vi "SMR_LabVIEW_V2.vi"() -> ()   [LabVIEW 2025]
uses:
  <vilib>/DAQmx/read.llb/DAQmx Read (Analog 1D DBL NChan 1Samp).vi
  <vilib>/Analysis/baseanly.llb/Mean (DBL).vi
  <vilib>/DAQmx/create/channels.llb/DAQmx Create Channel (AI-Temperature-Thermocouple).vi
  <vilib>/DAQmx/create/channels.llb/DAQmx Create Channel (AI-Voltage-Basic).vi
  <vilib>/DAQmx/miscellaneous.llb/DAQmx Fill In Error Info.vi
  <vilib>/Analysis/NI_AALBase.lvlib
panel:
  out "Raw NI9201 \nVoltage Display":T1
  out "Temperature Display":T2
  out "Pressure Display":T3
  in  "Flow Offset Correction (GPM)":dbl=-0.3
  out "Flow History":dbl(graph)
  out "Pressure History":T4(graph)
  out "Temperature History":T5(graph)
  out "Max Loop Pressure (psi)":dbl
  out "Average Loop Temp (deg C)":dbl
  out "Max Loop Temp (deg C)":dbl
  out "Heat Exchanger Flow (GPM)":dbl
  in  "Loop Period (ms)":dbl=1000.0
  in  "Stop":bool
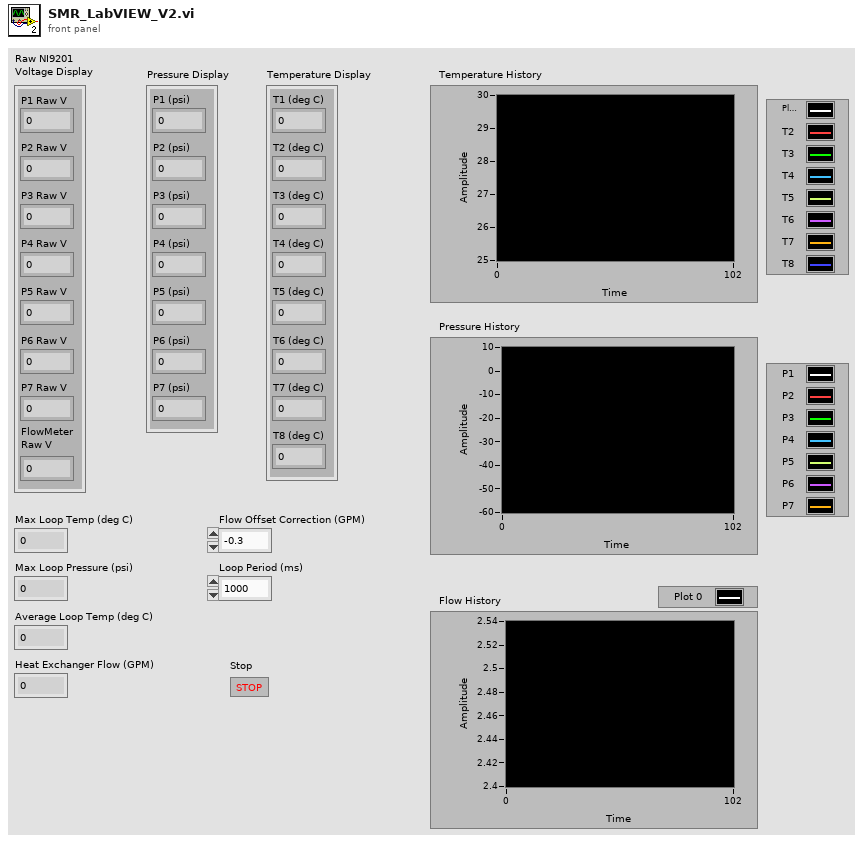
[diagram p1: front panel]
types:
  T1 = cluster{"P1 Raw V":dbl, "P2 Raw V":dbl, "P3 Raw V":dbl, "P4 Raw V":dbl, "P5 Raw V":dbl, "P6 Raw V":dbl, "P7 Raw V":dbl, "FlowMeter\nRaw V":dbl}
  T2 = cluster{"T1 (deg C)":dbl, "T2 (deg C)":dbl, "T3 (deg C)":dbl, "T4 (deg C)":dbl, "T5 (deg C)":dbl, "T6 (deg C)":dbl, "T7 (deg C)":dbl, "T8 (deg C)":dbl}
  T3 = cluster{"P1 (psi)":dbl, "P2 (psi)":dbl, "P3 (psi)":dbl, "P4 (psi)":dbl, "P5 (psi)":dbl, "P6 (psi)":dbl, "P7 (psi)":dbl}
  T4 = cluster{"P1":dbl, "P2":dbl, "P3":dbl, "P4":dbl, "P5":dbl, "P6":dbl, "P7":dbl}
  T5 = cluster{"Waveform":dbl, "Waveform":dbl, "Waveform":dbl, "Waveform":dbl, "Waveform":dbl, "Waveform":dbl, "Waveform":dbl, "Waveform":dbl}
  T6 = cluster{"P1":dbl, "P2":dbl, "P3":dbl, "P4":dbl, "P5":dbl, "P6":dbl, "P7":dbl, "Flow":dbl}
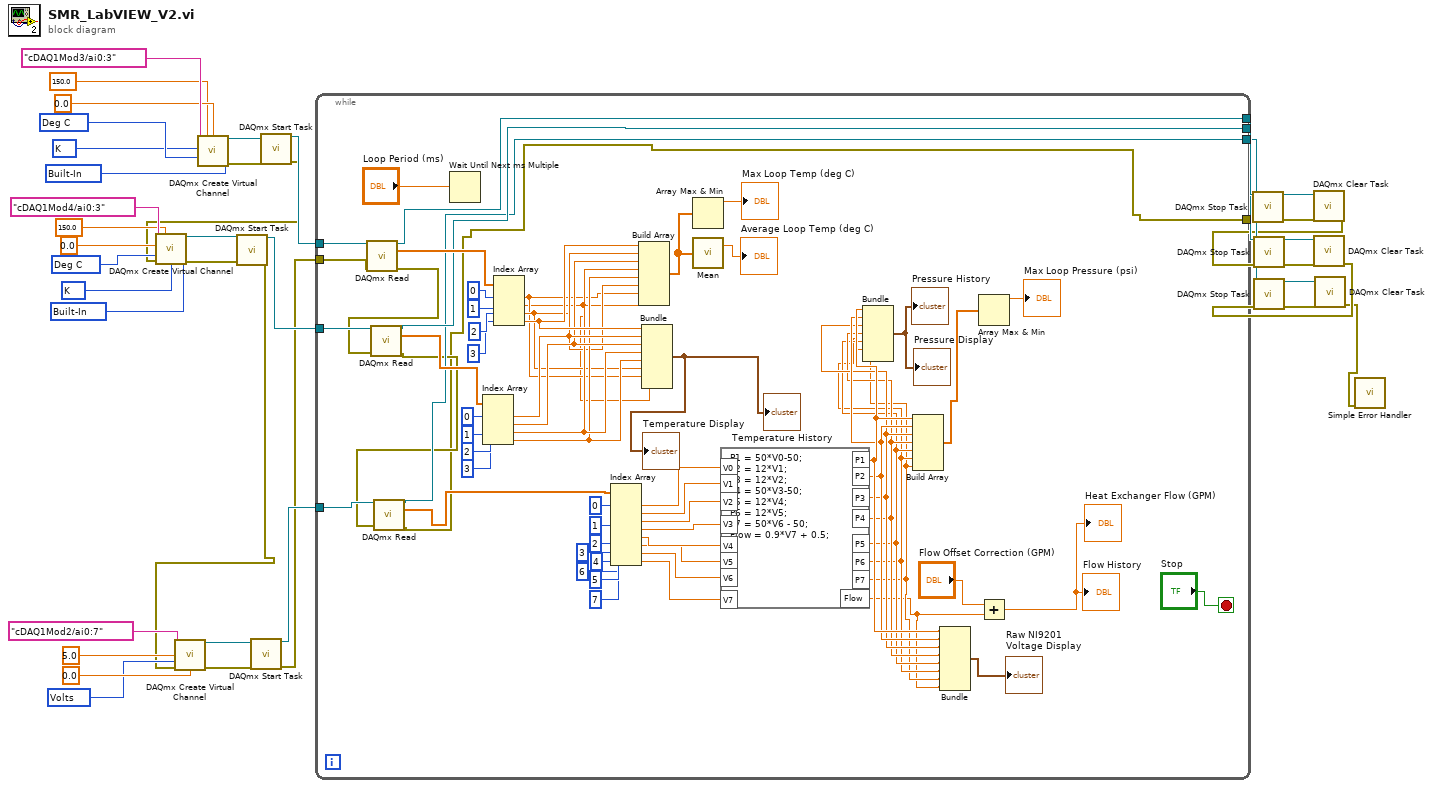
[diagram p0: block diagram]
diagram:
  w23 = 10348 items=["Volts"=10348, "From Custom Scale"=10065] ("units")
  w27 = 10200 items=["Built-In"=10200, "Constant Value"=10116, "Channel"=10113] ("cjc source")
  w28 = 10073 items=["J"=10072, "K"=10073, "N"=10077, "R"=10082, "S"=10085, "T"=10086, "B"=10047, "E"=10055] ("thermocouple type")
  w11 = 10143 items=["Deg C"=10143, "Deg F"=10144, "Kelvins"=10325, "Deg R"=10145, "From Custom Scale"=10065] ("units")
  w31 = 10200 items=["Built-In"=10200, "Constant Value"=10116, "Channel"=10113] ("cjc source")
  w32 = 10073 items=["J"=10072, "K"=10073, "N"=10077, "R"=10082, "S"=10085, "T"=10086, "B"=10047, "E"=10055] ("thermocouple type")
  w35 = 10143 items=["Deg C"=10143, "Deg F"=10144, "Kelvins"=10325, "Deg R"=10145, "From Custom Scale"=10065] ("units")
  n1 = call-poly <vilib>:"DAQmx Create Virtual Channel.vi"("maximum value"=150.0, "minimum value"=0.0, "physical channels"=tag "cDAQ1Mod3/ai0:3", "cjc source"=w31, "units"=w35, "thermocouple type"=w32) -> ("task out"=w40:refnum<k21>, "error out"=w39:errorcluster)  [unwired: 8 in]
  n2 = call <vilib>:"DAQmx Start Task.vi"("task/channels in"=w40, "error in"=w39) -> ("task out"=w20:refnum<k21>, "error out"=w10:errorcluster)  [unwired: 12 in]
  n3 = call-poly <vilib>:"DAQmx Create Virtual Channel.vi"("maximum value"=150.0, "minimum value"=0.0, "physical channels"=tag "cDAQ1Mod4/ai0:3", "cjc source"=w27, "units"=w11, "error in"=w10, "thermocouple type"=w28) -> ("task out"=w37:refnum<k21>, "error out"=w36:errorcluster)  [unwired: 7 in]
  n4 = call <vilib>:"DAQmx Start Task.vi"("task/channels in"=w37, "error in"=w36) -> ("task out"=w19:refnum<k21>, "error out"=w9:errorcluster)  [unwired: 12 in]
  n5 = call-poly <vilib>:"DAQmx Create Virtual Channel.vi"("maximum value"=5.0, "minimum value"=0.0, "physical channels"=tag "cDAQ1Mod2/ai0:7", "units"=w23, "error in"=w9) -> ("task out"=w22:refnum<k21>, "error out"=w21:errorcluster)  [unwired: 9 in]
  n6 = call <vilib>:"DAQmx Start Task.vi"("task/channels in"=w22, "error in"=w21) -> ("task out"=w18:refnum<k21>, "error out"=w8:errorcluster)  [unwired: 12 in]
  n7 = while {
    tunnel: w20 -> [w104]
    tunnel: w19 -> [w103]
    tunnel: w18 -> [w89]
    tunnel: [w70] -> w17
    tunnel: [w69] -> w16
    tunnel: [w68] -> w15
    tunnel: w8 -> [w67]
    tunnel: [w64] -> w7
    stop <- "Stop" stop-if-true
    n8 = call-poly <vilib>:"DAQmx Read.vi"("task/channels in"=w104, "error in"=w67) -> ("task out"=w70:refnum<k21>, "data"=w94:dbl[], "error out"=w66:errorcluster)  [unwired: 11 in]
    n9 = call-poly <vilib>:"DAQmx Read.vi"("task/channels in"=w103, "error in"=w66) -> ("task out"=w69:refnum<k21>, "data"=w93:dbl[], "error out"=w65:errorcluster)  [unwired: 11 in]
    n10 = call-poly <vilib>:"DAQmx Read.vi"("task/channels in"=w89, "error in"=w65) -> ("task out"=w68:refnum<k21>, "data"=w80:dbl[], "error out"=w64:errorcluster)  [unwired: 11 in]
    n11 = Wait Until Next ms Multiple(millisecond multiple="Loop Period (ms)") -> ()  [unwired: 1 out]
    n12 = Index Array(array=w93, index #1=0 ("index"), index #2=1 ("index"), index #3=2 ("index"), index #4=3 ("index")) -> (element #1=w62:dbl, element #2=w61:dbl, element #3=w60:dbl, element #4=w59:dbl)
    n13 = Index Array(array=w94, index #1=0 ("index"), index #2=1 ("index"), index #3=2 ("index"), index #4=3 ("index")) -> (element #1=w57:dbl, element #2=w56:dbl, element #3=w58:dbl, element #4=w63:dbl)
    n14 = Index Array(array=w80, index #1=0 ("index"), index #2=1 ("index"), index #3=2 ("index"), index #4=3 ("index"), index #5=4 ("index"), index #6=5 ("index"), index #7=6 ("index"), index #8=7 ("index")) -> (element #1=w79:dbl, element #2=w78:dbl, element #3=w77:dbl, element #4=w76:dbl, element #5=w75:dbl, element #6=w74:dbl, element #7=w73:dbl, element #8=w72:dbl)
    n15 = Build Array(w63, w62, w61, w60, w59, w58, w57, w56) -> (w91:dbl[])
    n16 = Bundle("Waveform"=w63, "Waveform"=w62, "Waveform"=w61, "Waveform"=w60, "Waveform"=w59, "Waveform"=w58, "Waveform"=w57, "Waveform"=w56) -> (→"Temperature History" →"Temperature Display":T5)  [unwired: 1 in]
    n17 = Array Max & Min(array=w91) -> (max value=→"Max Loop Temp (deg C)":dbl)  [unwired: 3 out]
    n18 = call-poly <vilib>:"Mean.vi"("X"=w91) -> ("mean"=→"Average Loop Temp (deg C)":dbl)  [unwired: 1 out]
    n19 = formula code="P1 = 50*V0-50;\nP2 = 12*V1;\nP3 = 12*V2;\nP4 = 50*V3-50;\nP5 = 12*V4;\nP6 = 12*V5; \nP7 = 50*V6 - 50;\nFlow = 0.9*V7 + 0.5;"("V0"=w79, "V1"=w78, "V2"=w77, "V3"=w76, "V4"=w75, "V5"=w74, "V6"=w73, "V7"=w72) -> ("P1"=w50:dbl, "P2"=w49:dbl, "P3"=w48:dbl, "P4"=w47:dbl, "P5"=w46:dbl, "P6"=w45:dbl, "P7"=w44:dbl, "Flow"=w43:dbl)
    n20 = Bundle("P1"=w50, "P2"=w49, "P3"=w48, "P4"=w47, "P5"=w46, "P6"=w45, "P7"=w44) -> (→"Pressure History" →"Pressure Display":T4)  [unwired: 1 in]
    n21 = Build Array(w50, w49, w48, w47, w46, w45, w44) -> (w53:dbl[])
    n22 = Bundle("P1"=w50, "P2"=w49, "P3"=w48, "P4"=w47, "P5"=w46, "P6"=w45, "P7"=w44, "Flow"=w43) -> (→"Raw NI9201 \nVoltage Display":T6)  [unwired: 1 in]
    n23 = Array Max & Min(array=w53) -> (max value=→"Max Loop Pressure (psi)":dbl)  [unwired: 3 out]
    n24 = Add(x="Flow Offset Correction (GPM)", y=w43) -> (x+y=→"Heat Exchanger Flow (GPM)" →"Flow History":dbl)
  }
  n25 = call <vilib>:"DAQmx Stop Task.vi"("task/channels in"=w17, "error in"=w7) -> ("task out"=w14:refnum<k21>, "error out"=w6:errorcluster)  [unwired: 12 in]
  n26 = call <vilib>:"DAQmx Clear Task.vi"("task in"=w14, "error in"=w6) -> ("error out"=w5:errorcluster)  [unwired: 13 in]
  n27 = call <vilib>:"DAQmx Stop Task.vi"("task/channels in"=w16, "error in"=w5) -> ("task out"=w13:refnum<k21>, "error out"=w4:errorcluster)  [unwired: 12 in]
  n28 = call <vilib>:"DAQmx Clear Task.vi"("task in"=w13, "error in"=w4) -> ("error out"=w3:errorcluster)  [unwired: 13 in]
  n29 = call <vilib>:"DAQmx Stop Task.vi"("task/channels in"=w15, "error in"=w3) -> ("task out"=w12:refnum<k21>, "error out"=w2:errorcluster)  [unwired: 12 in]
  n30 = call <vilib>:"DAQmx Clear Task.vi"("task in"=w12, "error in"=w2) -> ("error out"=w1:errorcluster)  [unwired: 13 in]
  n31 = call <vilib>:"Simple Error Handler.vi"("error in (no error)"=w1) -> ()  [unwired: 4 in, 5 out]
